vi "All Data.vi"() -> ()   [LabVIEW 2020]
uses:
  Libraries/Packages/Repo_class/Repo.lvclass/Repo.ctl
  Libraries/Packages/Package_class/Package.lvclass/Package.ctl
  Libraries/Packages/Package Version_class/Package Version.lvclass/Package Version.ctl
  Libraries/Packages/Package_class/Read DisplayName.vi
  Libraries/Packages/Package_class/Read Name.vi
  Libraries/Packages/Package_class/Read RepoName.vi
  Libraries/Packages/Package_class/Read RepoType.vi
  Libraries/Packages/Package_class/Read Versions.vi
  Libraries/Packages/Package Version_class/Read Author.vi
  Libraries/Packages/Package Version_class/Read Dependencies.vi
  Libraries/Packages/Package Version_class/Read Description.vi
  Libraries/Packages/Package Version_class/Read DisplayName.vi
  Libraries/Packages/Package Version_class/Read IconURL.vi
  Libraries/Packages/Package Version_class/Read Name.vi
  Libraries/Packages/Package Version_class/Read PackageURL.vi
  Libraries/Packages/Package Version_class/Read Release Notes.vi
  Libraries/Packages/Package Version_class/Read ReleaseDate.vi
  Libraries/Packages/Package Version_class/Read RepoName.vi
  Libraries/Packages/Package Version_class/Read RepoType.vi
  Libraries/Packages/Package Version_class/Read Vendor.vi
  Libraries/Packages/Package Version_class/Read Version.vi
  Libraries/Packages/Package Version_class/Read Summary.vi
  Libraries/Packages/Repo_class/Read LastUpdated.vi
  Libraries/Packages/Repo_class/Read Name.vi
  Libraries/Packages/Repo_class/Read RepoType.vi
  Libraries/Packages/Repo_class/Read URL.vi
  Libraries/Packages/Repo_class/Read Packages.vi
  Libraries/Packages/Package_class/Package.lvclass
  Libraries/Packages/Package Version_class/Package Version.lvclass
  Libraries/WSsupport/WSsupport.lvlib
  Libraries/Packages/Repo_class/Repo.lvclass
panel:
  out "spreadsheet string":string
  out "size(s)":i32[](array[numeric])
  in  "Multicolumn Listbox":i32(listbox)
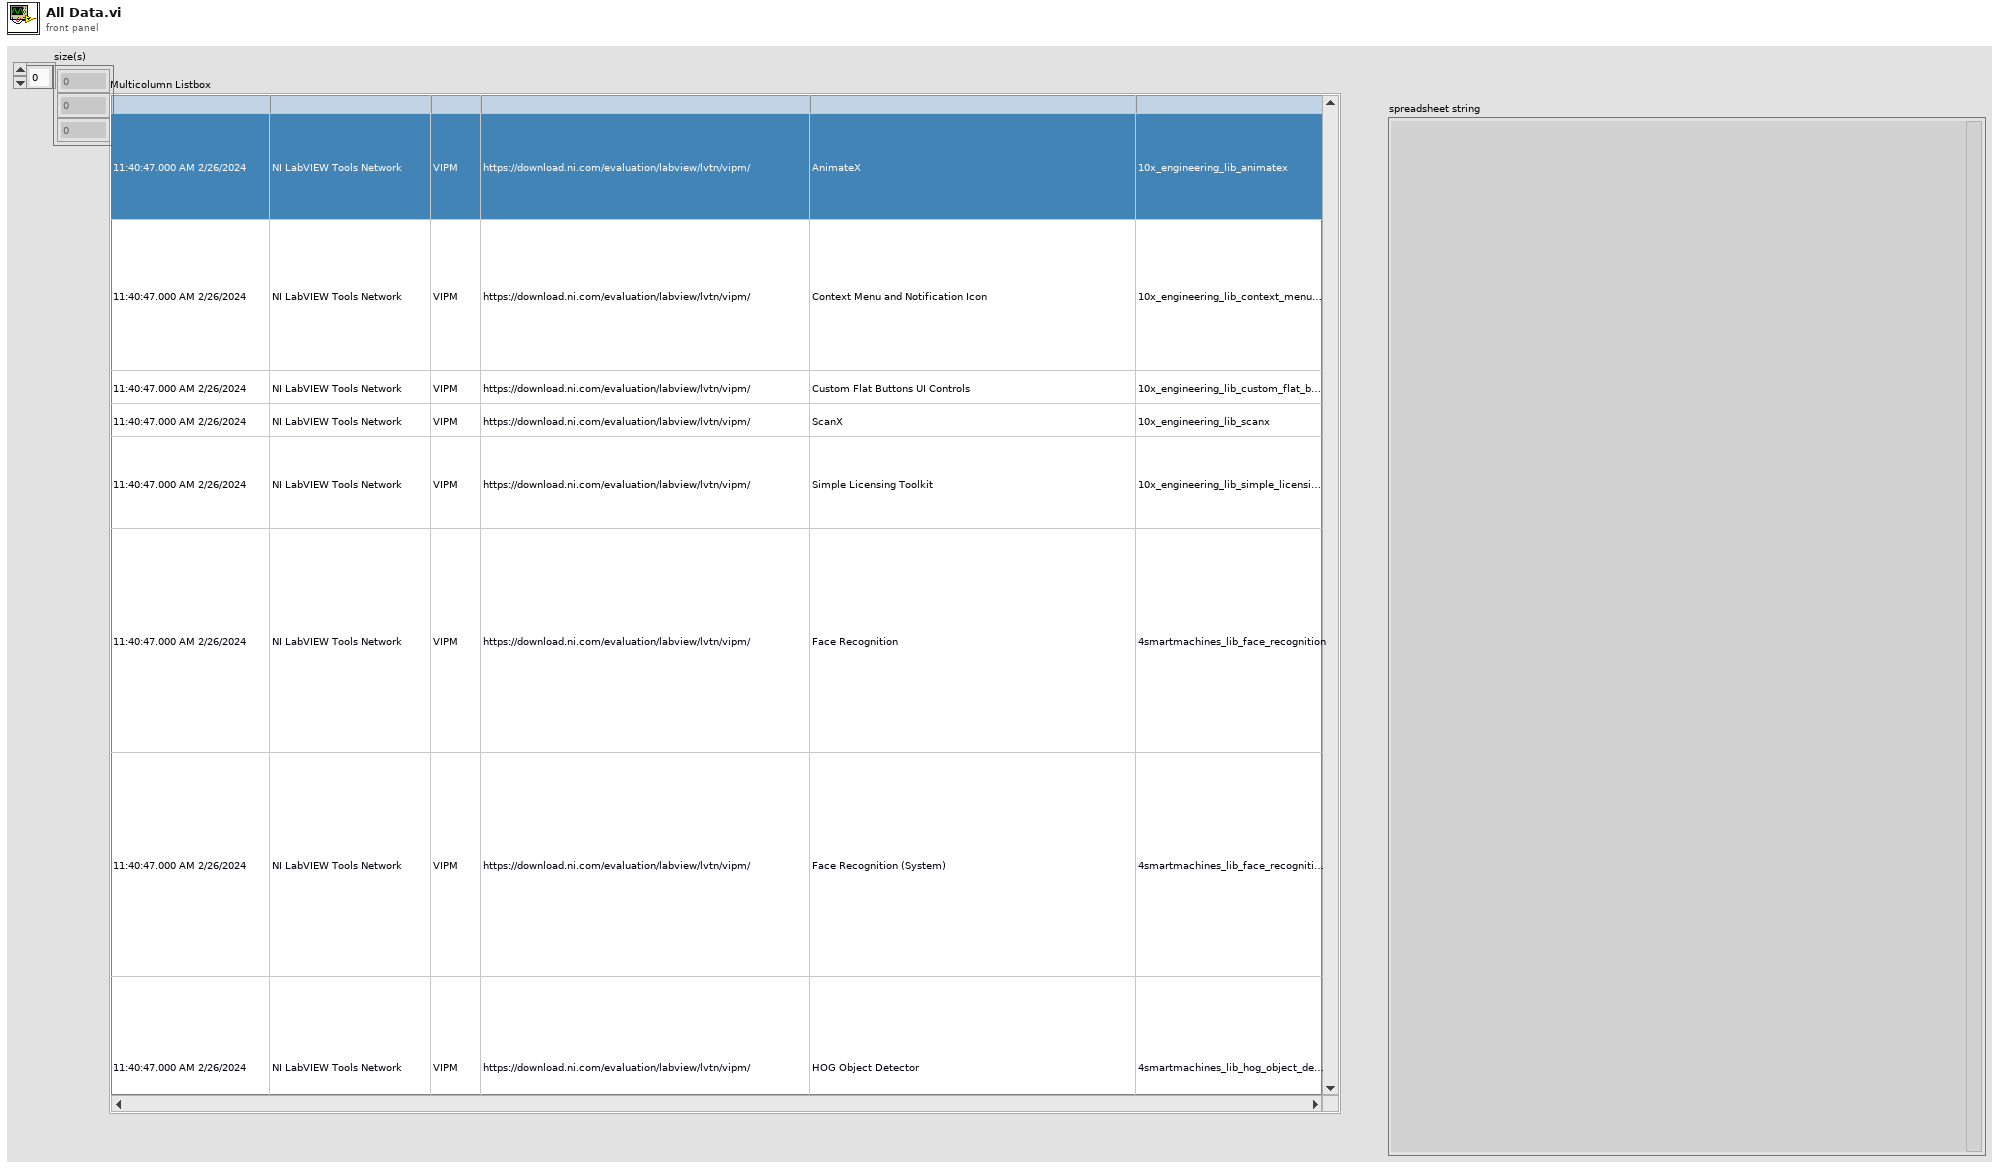
[diagram p1: front panel]
types:
  T1 = typedef "Packages.lvlib/Repo.lvclass/RepoType--enum.ctl" = enum16{"VIPM", "NIPM", "GPM"}
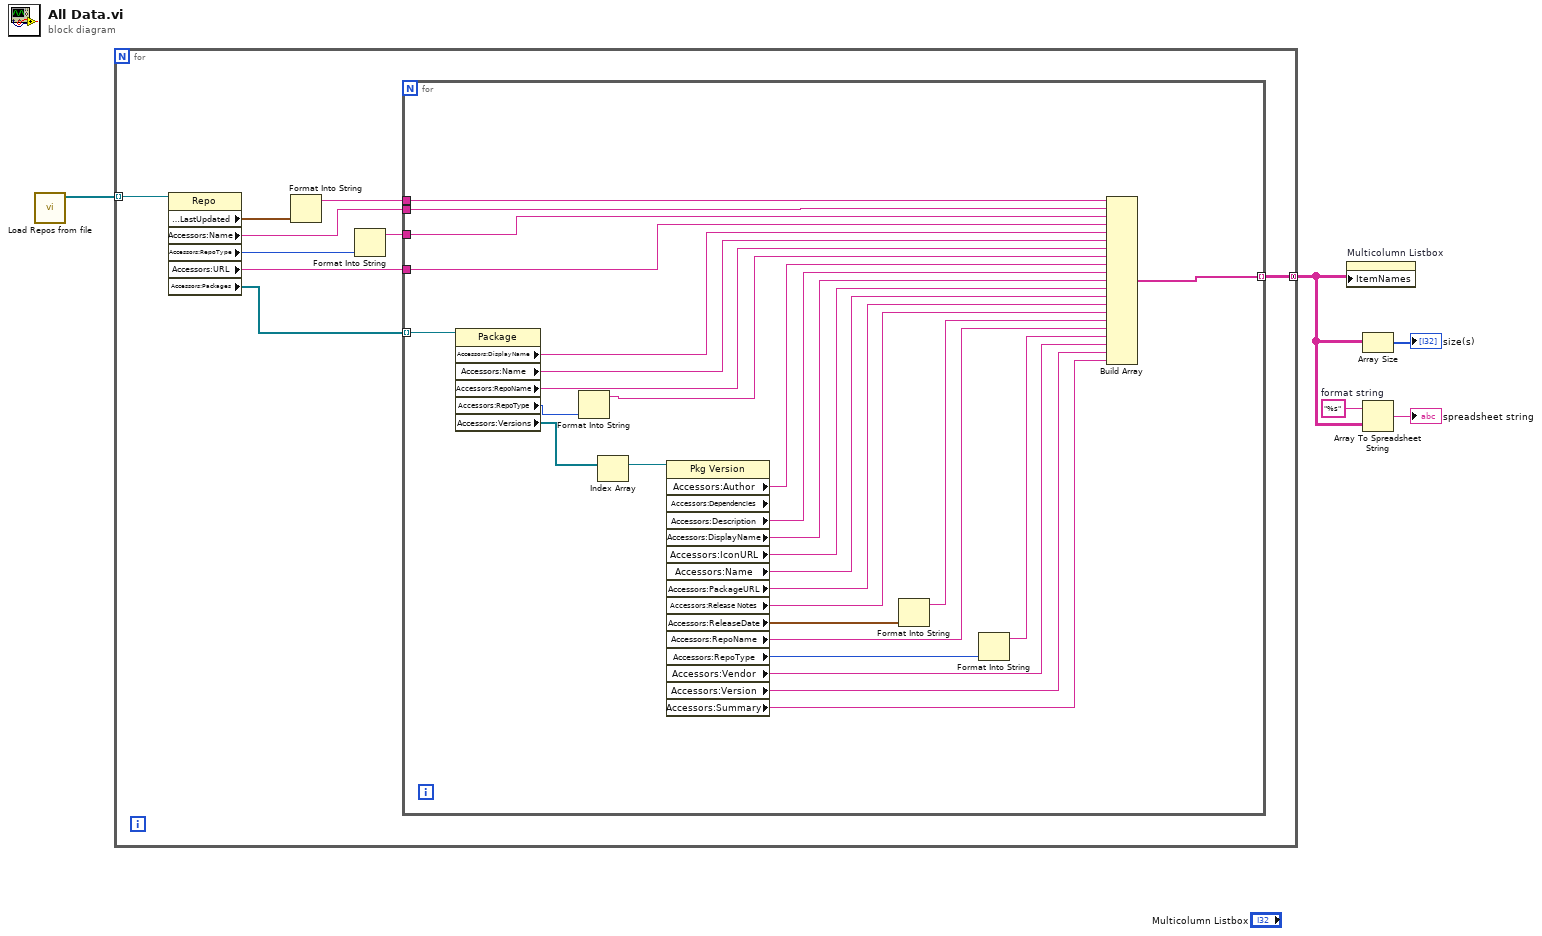
[diagram p0: block diagram]
diagram:
  w2 = "%s"  # format string
  n1 = call "Load Repos from file.vi"() -> ("Repos"=w5:refnum<class "Repo.lvclass">[])  [unwired: 10 in, 1 out]
  n2 = for {
    tunnel: w5 -> [w14] mode=indexing
    tunnel: [w6] -> w3 mode=concatenating
    n3 = property class="Repo"(reference=w14) -> ("Accessors:LastUpdated"=w13:timestamp, "Accessors:Name"=w9:string, "Accessors:RepoType"=w12:T1, "Accessors:URL"=w7:string, "Accessors:Packages"=w11:refnum<class "Package.lvclass">[])  [unwired: 1 in, 2 out]
    n4 = Format Into String(w13) -> (resulting string=w10:string)  [unwired: 3 in, 1 out]
    n5 = Format Into String(w12) -> (resulting string=w8:string)  [unwired: 3 in, 1 out]
    n6 = for {
      tunnel: w11 -> [w42] mode=indexing
      tunnel: w10 -> [w39]
      tunnel: w9 -> [w38]
      tunnel: w8 -> [w37]
      tunnel: w7 -> [w36]
      tunnel: [w31] -> w6 mode=indexing
      n7 = property class="Package"(reference=w42) -> ("Accessors:DisplayName"=w35:string, "Accessors:Name"=w34:string, "Accessors:RepoName"=w33:string, "Accessors:RepoType"=w40:T1, "Accessors:Versions"=w41:refnum<class "Package Version.lvclass">[])  [unwired: 1 in, 2 out]
      n8 = Format Into String(w40) -> (resulting string=w32:string)  [unwired: 3 in, 1 out]
      n9 = Index Array(array=w41) -> (element=w16:refnum<class "Package Version.lvclass">)  [unwired: 1 in]
      n10 = property class="Pkg Version" props=["Accessors:Author", "Accessors:Dependencies", "Accessors:Description", "Accessors:DisplayName", "Accessors:IconURL", "Accessors:Name", "Accessors:PackageURL", "Accessors:Release Notes", "Accessors:ReleaseDate", "Accessors:RepoName", "Accessors:RepoType", "Accessors:Vendor", "Accessors:Version", "Accessors:Summary"](reference=w16) -> ("Accessors:Author"=w30:string, "Accessors:Description"=w29:string, "Accessors:DisplayName"=w28:string, "Accessors:IconURL"=w26:string, "Accessors:Name"=w25:string, "Accessors:PackageURL"=w24:string, "Accessors:Release Notes"=w23:string, "Accessors:ReleaseDate"=w27:timestamp, "Accessors:RepoName"=w21:string, "Accessors:RepoType"=w20:T1, "Accessors:Vendor"=w18:string, "Accessors:Version"=w17:string, "Accessors:Summary"=w15:string)  [unwired: 1 in, 3 out]
      n11 = Format Into String(w27) -> (resulting string=w22:string)  [unwired: 3 in, 1 out]
      n12 = Format Into String(w20) -> (resulting string=w19:string)  [unwired: 3 in, 1 out]
      n13 = Build Array(w39, w38, w37, w36, w35, w34, w33, w32, w30, w29, w28, w26, w25, w24, w23, w22, w21, w19, w18, w17, w15) -> (w31:string[])
    }
  }
  n14 = property on="Multicolumn Listbox" class="MCListbox (strict)"("ItemNames"=w3) -> ()  [unwired: 2 in, 2 out]
  n15 = Array Size(array=w3) -> (size(s)=→"size(s)":i32[])
  n16 = Array To Spreadsheet String(array=w3, 3:w2) -> (spreadsheet string=→"spreadsheet string":string)  [unwired: 1 in]
